vi "Cal Inst Control.vi"(8 "error in (no error)":errorcluster, 10 "Master":refnum<queue>, 11 "Sub Panel ref":refnum<vi>) -> (0 "error out":errorcluster)   [LabVIEW 2014, in "Instrument Launcher.lvlib"]
uses:
  CaliforniaInstrumentsIxSeries/support/Message Queue/Message Cluster.ctl
  Instrument Launcher.lvlib
  CaliforniaInstrumentsIxSeries/support/Message Queue/Cal Inst Message Queue.lvlib
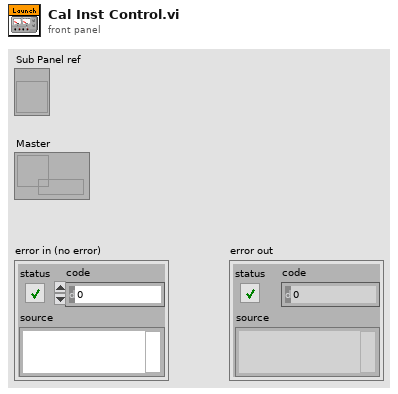
[diagram p1: front panel]
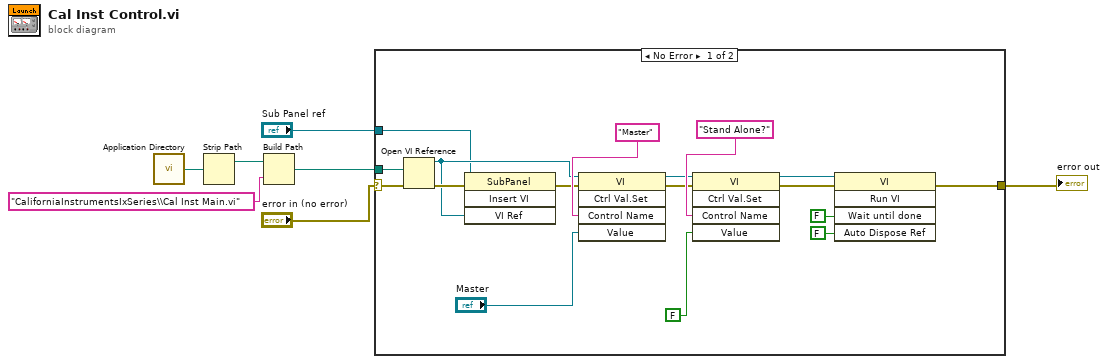
[diagram p0: block diagram]
diagram:
  n1 = call <vilib>:"Application Directory.vi"() -> ("Application Directory"=w3:path)
  n2 = Strip Path(path=w3) -> (stripped path=w2:path)  [unwired: 1 out]
  n3 = Build Path(base path=w2, name or relative path="CaliforniaInstrumentsIxSeries\\Cal Inst Main.vi") -> (appended path=w1:path)
  n4 = case shown="No Error" "error in (no error)" {
    selector: "error in (no error)" -> [w8 w25]
    tunnel: [w16 w25] -> w7
    tunnel: w1 -> [w14 _]
    tunnel: "Sub Panel ref" -> [w11 _]
    frame No Error {
      n5 = Open VI Reference(vi path=w14, error in (no error)=w8) -> (vi reference=w12:refnum<vi>, error out=w15:errorcluster)  [unwired: 4 in]
      n6 = invoke on="Invoke Node" class="SubPanel" method="Insert VI"(reference=w11, error in=w15, "VI Ref"=w12) -> (error out=w13:errorcluster)  [unwired: 1 in, 3 out]
      n7 = invoke class="VI" method="Ctrl Val.Set"(reference=w12, error in=w13, "Control Name"="Master", "Value"="Master") -> (reference out=w10:refnum<vi>, error out=w9:errorcluster)  [unwired: 1 in, 3 out]
      n8 = invoke class="VI" method="Ctrl Val.Set"(reference=w10, error in=w9, "Control Name"="Stand Alone?", "Value"=FALSE) -> (reference out=w20:refnum<vi>, error out=w19:errorcluster)  [unwired: 1 in, 3 out]
      n9 = invoke class="VI" method="Run VI"(reference=w20, error in=w19, "Wait until done"=FALSE ("Wait Until Done"), "Auto Dispose Ref"=FALSE ("Auto Dispose Reference")) -> (error out=w16:errorcluster)  [unwired: 1 in, 4 out]
    }
    frame Error {
    }
  }
  "error out" <- w7
